vi "Read Config from File.vi"(8 "error in":errorcluster, 11 "Config File":path) -> (0 "error out":errorcluster, 2 "Configuration":T1)   [LabVIEW 2020, in "cycling structure demo UI.lvlib" / "Configuration.lvclass"]
doc: "Read the configuration from file.\n____\nPeloton Config 2.0.0.6\nCopyright (c) 2024, Peloton"
uses:
  Configuration.lvclass
  Configuration--cluster.ctl
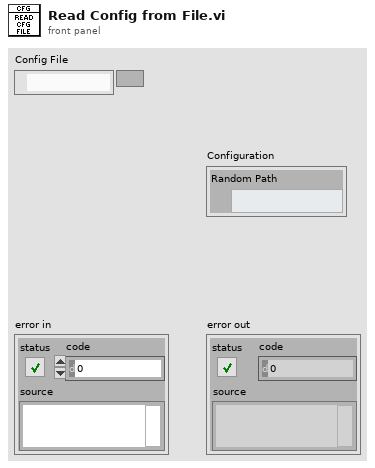
[diagram p1: front panel]
types:
  T1 = typedef "cycling structure demo UI.lvlib/Configuration.lvclass/Configuration--cluster.ctl" = cluster{"Random Path":path}
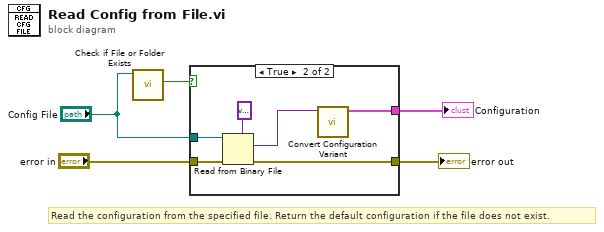
[diagram p0: block diagram]
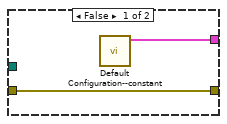
[diagram p2: hidden frame]
diagram:
  # "Read the configuration from the specified file. Return the default configuration if the file does not exist."
  n1 = call <vilib>:"Check if File or Folder Exists.vi"("path"="Config File") -> ("file or folder exists?"=w1:bool)  [unwired: 8 in, 2 out]
  n2 = case shown="True" w1 {
    tunnel: "error in" -> [w7 w13]
    tunnel: [w7 w12] -> w4
    tunnel: [w6 w9] -> w3
    tunnel: "Config File" -> [_ w8]
    frame False {
      n3 = call "Default Configuration--constant.vi"() -> ("Default Configuration"=w6:T1)  [unwired: 11 in]
    }
    frame True {
      n4 = Read from Binary File(5:variant, 8:w13, 11:w8) -> (0:w12:errorcluster, 2:w10:variant)  [unwired: 3 in, 2 out]
      n5 = call "Convert Configuration Variant.vi"("Current Configuration"=w10) -> ("Configuration"=w9:T1)  [unwired: 8 in, 2 out]
    }
  }
  "Configuration" <- w3
  "error out" <- w4
